vi "Update State.vi"(8 "error in (no error)":errorcluster, 9 "Digital Inputs":T1, 10 "Analog Inputs":T2, 11 "GripsMaster in":refnum<class "GripsMaster.lvclass">) -> (0 "error out":errorcluster, 3 "GripsMaster out":refnum<class "GripsMaster.lvclass">)   [LabVIEW 2011, in "GripsMaster.lvclass"]
uses:
  GripsMaster.lvclass
  controls/Analog Values.ctl
  controls/Digital Values.ctl
  GripsMaster.lvclass/GripsMaster.ctl
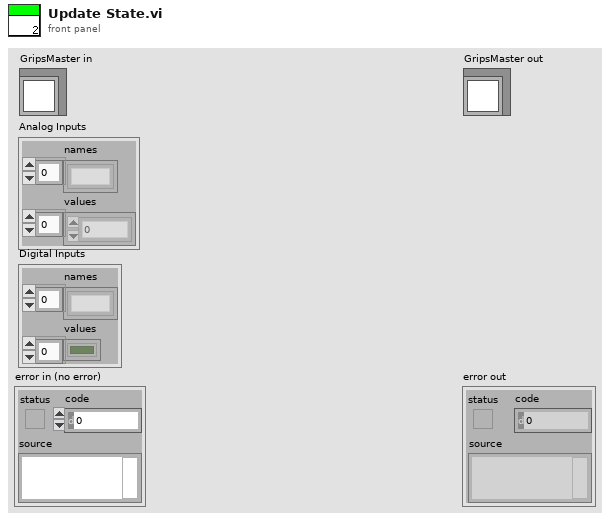
[diagram p1: front panel]
types:
  T1 = typedef "Digital Values.ctl" = cluster{"names":string[], "values":bool[]}
  T2 = typedef "Analog Values.ctl" = cluster{"names":string[], "values":dbl[]}
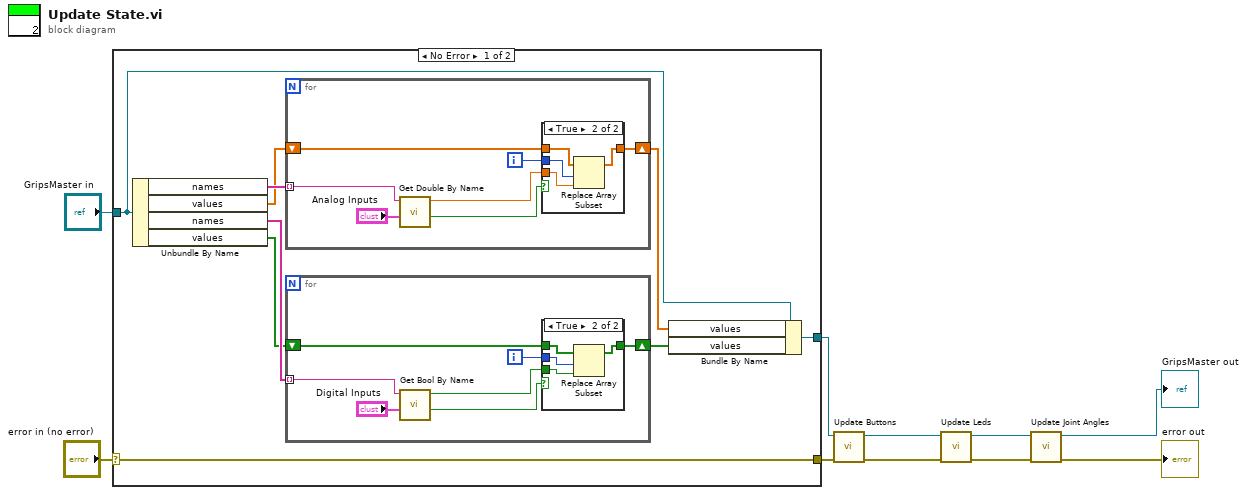
[diagram p0: block diagram]
diagram:
  n1 = case shown="No Error" "error in (no error)" {
    selector: "error in (no error)" -> [w19 w45]
    tunnel: [w19 w45] -> w7
    tunnel: [w18 w44] -> w8
    tunnel: "GripsMaster in" -> [w17 w44]
    frame No Error {
      n2 = Unbundle By Name(w17) -> ("names"=w16:string[], "values"=w15:dbl[], "names"=w13:string[], "values"=w12:bool[])
      n3 = for {
        tunnel: w16 -> [w37] mode=indexing
        shift-right: [w38] -> w14
        shift-left: w15 -> [w36]
        i -> [w35]
        n4 = call "Get Double By Name.vi"("name"=w37, "Analog Values"="Analog Inputs") -> ("result"=w33:dbl, "found?"=w34:bool)  [unwired: 7 in]
        n5 = case shown="True" w34 {
          tunnel: [w39 w43] -> w38
          tunnel: w36 -> [w39 w42]
          tunnel: w35 -> [_ w41]
          tunnel: w33 -> [_ w40]
          frame False {
          }
          frame True {
            n6 = Replace Array Subset(array=w42, new element=w40, index=w41) -> (w43:dbl[])
          }
        }
      }
      n7 = for {
        tunnel: w13 -> [w26] mode=indexing
        shift-right: [w21] -> w11
        shift-left: w12 -> [w23]
        i -> [w22]
        n8 = call "Get Bool By Name.vi"("name"=w26, "Digital Values"="Digital Inputs") -> ("result"=w24:bool, "found?"=w25:bool)  [unwired: 7 in]
        n9 = case shown="True" w25 {
          tunnel: [w27 w31] -> w21
          tunnel: w24 -> [_ w28]
          tunnel: w22 -> [_ w30]
          tunnel: w23 -> [w27 w29]
          frame False {
          }
          frame True {
            n10 = Replace Array Subset(array=w29, new element=w28, index=w30) -> (w31:bool[])
          }
        }
      }
      n11 = Bundle By Name(cluster=w17, "values"=w14, "values"=w11) -> (w18:refnum<class "GripsMaster.lvclass">)
    }
    frame Error {
    }
  }
  n12 = call "Update Buttons.vi"("error in (no error)"=w7, "GripsMaster in"=w8) -> ("error out"=w3:errorcluster, "GripsMaster out"=w4:refnum<class "GripsMaster.lvclass">)  [unwired: 8 in]
  n13 = call "Update Leds.vi"("error in (no error)"=w3, "GripsMaster in"=w4) -> ("error out"=w1:errorcluster, "GripsMaster out"=w2:refnum<class "GripsMaster.lvclass">)  [unwired: 8 in]
  n14 = call "Update Joint Angles.vi"("error in (no error)"=w1, "GripsMaster in"=w2) -> ("error out"=→"error out":errorcluster, "GripsMaster out"=→"GripsMaster out":refnum<class "GripsMaster.lvclass">)  [unwired: 8 in]
